vi "测量数据区.vi"(11 "数组":u16[](array[numeric]) format="%04xH") -> (3 "测量数据区":T1 {"单位" items=["ug/L", "mg/L", "ppm", "mg/m3", "cm", "ppb", "ug/m3", "%", "nmol/mol", "umol/mol", "MPN/L", "MPN/100ml", "ng/m3", "NTU", "无量纲", "ms/cm", "us/cm", "℃", "mV", "万个/L"]})   [LabVIEW 2016, in "质控单元V1.lvlib"]
panel:
  # "共占用82 WORD"
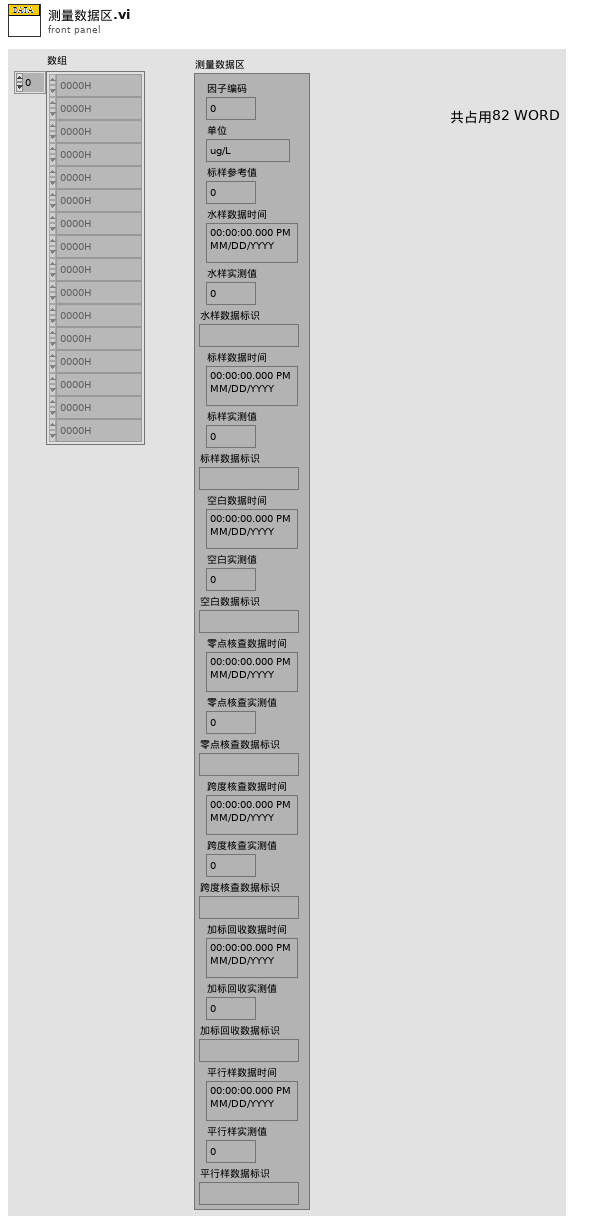
[diagram p1: front panel]
types:
  T1 = cluster{"因子编码":u32, "单位":u16, "标样参考值":sgl, "水样数据时间":timestamp, "水样实测值":sgl, "水样数据标识":string, "标样数据时间":timestamp, "标样实测值":sgl, "标样数据标识":string, "空白数据时间":timestamp, "空白实测值":sgl, "空白数据标识":string, "零点核查数据时间":timestamp, "零点核查实测值":sgl, "零点核查数据标识":string, "跨度核查数据时间":timestamp, "跨度核查实测值":sgl, "跨度核查数据标识":string, "加标回收数据时间":timestamp, "加标回收实测值":sgl, "加标回收数据标识":string, "平行样数据时间":timestamp, "平行样实测值":sgl, "平行样数据标识":string}
  T2 = cluster{"DWORD":i32, "WORD":u16, "FLOAT":sgl, "time stamp":timestamp, "数值":sgl, "string":string, "time stamp":timestamp, "数值":sgl, "string":string, "time stamp":timestamp, "数值":sgl, "string":string, "time stamp":timestamp, "数值":sgl, "string":string, "time stamp":timestamp, "数值":sgl, "string":string, "time stamp":timestamp, "数值":sgl, "string":string, "time stamp":timestamp, "数值":sgl, "string":string}
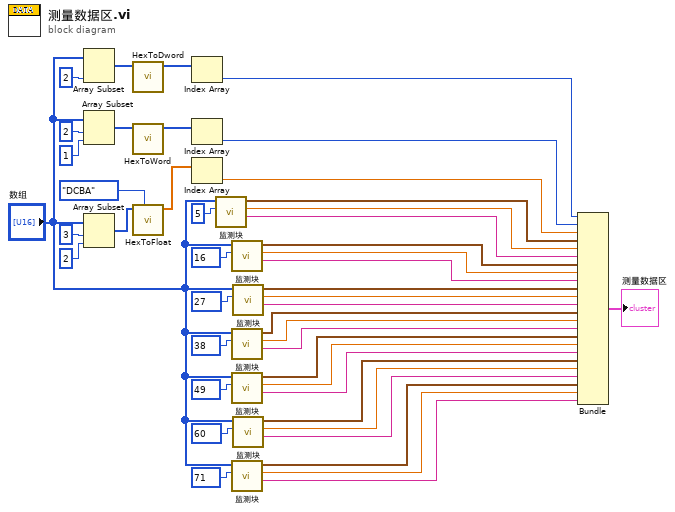
[diagram p0: block diagram]
diagram:
  n1 = Array Subset(array="数组", length=2 ("长度")) -> (w45:u16[])  [unwired: 1 in]
  n2 = Array Subset(array="数组", index=2 ("索引"), length=1 ("长度")) -> (w40:u16[])
  n3 = Array Subset(array="数组", index=3 ("索引"), length=2 ("长度")) -> (w35:u16[])
  n4 = call "HexToDword.vi"("数组"=w45) -> ("DWORD"=w43:i32[])  [unwired: 10 in]
  n5 = call "HexToWord.vi"("数组"=w40) -> ("WORD"=w39:u16[])  [unwired: 10 in]
  n6 = call "HexToFloat.vi"("转换类型"=enum16{"DCBA", "CDAB"}."DCBA", "数组"=w35) -> ("FLOAT"=w34:sgl[])  [unwired: 9 in]
  n7 = Index Array(array=w43) -> (element=w4:i32)  [unwired: 1 in]
  n8 = Index Array(array=w39) -> (element=w38:u16)  [unwired: 1 in]
  n9 = Index Array(array=w34) -> (element=w33:sgl)  [unwired: 1 in]
  n10 = call "监测块.vi"("索引"=5, "数组"="数组") -> ("string"=w30:string, "数值"=w31:sgl, "time stamp"=w32:timestamp)  [unwired: 7 in]
  n11 = call "监测块.vi"("索引"=16, "数组"="数组") -> ("string"=w25:string, "数值"=w26:sgl, "time stamp"=w27:timestamp)  [unwired: 7 in]
  n12 = call "监测块.vi"("索引"=38, "数组"="数组") -> ("string"=w17:string, "数值"=w18:sgl, "time stamp"=w19:timestamp)  [unwired: 7 in]
  n13 = call "监测块.vi"("索引"=49, "数组"="数组") -> ("string"=w13:string, "数值"=w14:sgl, "time stamp"=w15:timestamp)  [unwired: 7 in]
  n14 = call "监测块.vi"("索引"=71, "数组"="数组") -> ("string"=w5:string, "数值"=w6:sgl, "time stamp"=w7:timestamp)  [unwired: 7 in]
  n15 = call "监测块.vi"("索引"=27, "数组"="数组") -> ("string"=w21:string, "数值"=w22:sgl, "time stamp"=w23:timestamp)  [unwired: 7 in]
  n16 = call "监测块.vi"("索引"=60, "数组"="数组") -> ("string"=w9:string, "数值"=w10:sgl, "time stamp"=w11:timestamp)  [unwired: 7 in]
  n17 = Bundle("DWORD"=w4, "WORD"=w38, "FLOAT"=w33, "time stamp"=w32, "数值"=w31, "string"=w30, "time stamp"=w27, "数值"=w26, "string"=w25, "time stamp"=w23, "数值"=w22, "string"=w21, "time stamp"=w19, "数值"=w18, "string"=w17, "time stamp"=w15, "数值"=w14, "string"=w13, "time stamp"=w11, "数值"=w10, "string"=w9, "time stamp"=w7, "数值"=w6, "string"=w5) -> (→"测量数据区":T2)  [unwired: 1 in]
